vi "EEI EXP2.vi"() -> ()   [LabVIEW 2020]
panel:
  in  "y":dbl
  in  "x":dbl
  out "boolean output 2":bool
  in  "x":dbl
  out "boolean output":bool
  out "current time":timestamp
  out "result 2":bool
  in  "Binary input 6":bool
  in  "Binary input 5":bool
  in  "Binary input 4":bool
  out "result":bool
  in  "Binary input 3":bool
  in  "Binary input 2":bool
  in  "Binary input 1":bool
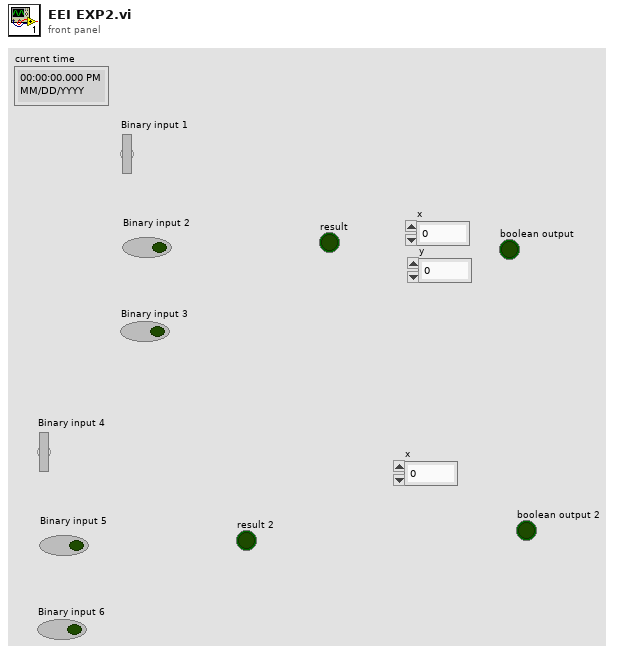
[diagram p1: front panel]
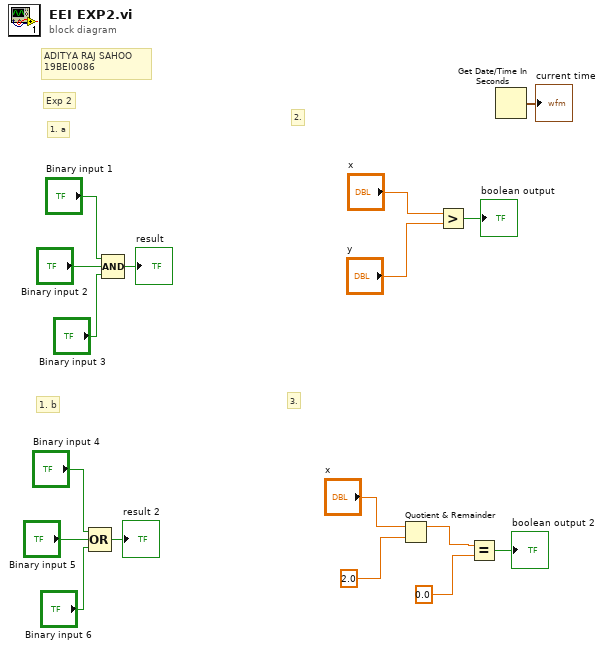
[diagram p0: block diagram]
diagram:
  # "ADITYA RAJ SAHOO\n19BEI0086"
  # "3."
  # "2."
  # "1. b"
  # "1. a"
  # "Exp 2"
  n1 = Compound Arithmetic op=OR("Binary input 4", "Binary input 5", "Binary input 6") -> (→"result 2":bool)
  n2 = Compound Arithmetic op=AND("Binary input 1", "Binary input 2", "Binary input 3") -> (→"result":bool)
  n3 = Quotient & Remainder(x="x", y=2.0) -> (x-y*floor(x/y)=w5:dbl)  [unwired: 1 out]
  n4 = Greater?(x="x", y="y") -> (0:→"boolean output":bool)
  n5 = Equal?(x=w5, y=0.0) -> (x = y?=→"boolean output 2":bool)
  n6 = Get Date/Time In Seconds() -> (seconds since 1Jan1904=→"current time":timestamp)
